vi "Row_Sum.vi"(0 "Image_2d":i16[][](array[numeric]), 5 "error in (no error)":errorcluster) -> (14 "Row_Sum":i16[](array[numeric]), 19 "error out":errorcluster)   [LabVIEW 2016]
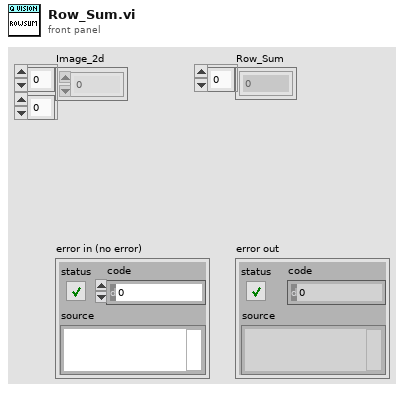
[diagram p1: front panel]
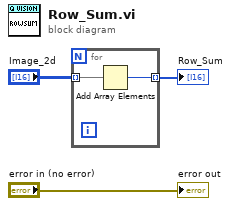
[diagram p0: block diagram]
diagram:
  n1 = for {
    tunnel: "Image_2d" -> [w5] mode=indexing
    tunnel: [w4] -> w3 mode=indexing
    n2 = Add Array Elements(numeric array=w5) -> (sum=w4:i16)
  }
  "Row_Sum" <- w3
  "error out" <- "error in (no error)"
